vi "Run_Core.vi"(0 "Message Popup in":refnum<class "ControllerData.lvclass">, 11 "error in (no error)":errorcluster) -> (4 "Message Popup out":refnum<class "ControllerData.lvclass">, 6 "Return":variant, 15 "error out":errorcluster)   [LabVIEW 2019, in "ControllerData.lvclass"]
uses:
  ControllerData.lvclass
  ControllerData.lvclass/ControllerData.ctl
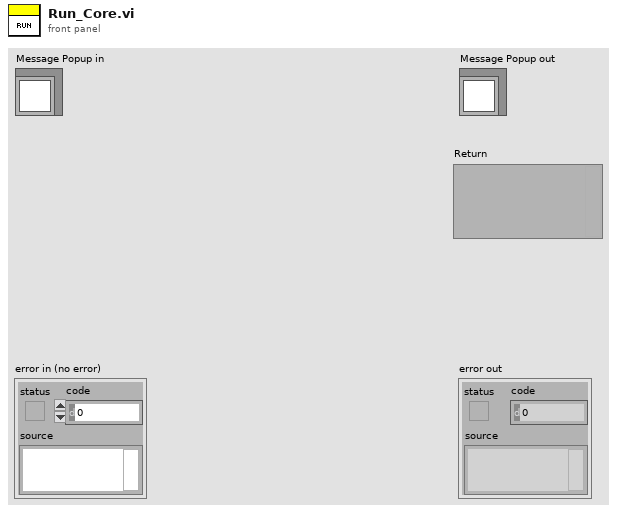
[diagram p1: front panel]
types:
  T1 = typedef "ControllerData.lvclass/Function List.ctl" = enum16{"GetTempTrend", "GetStatus"}
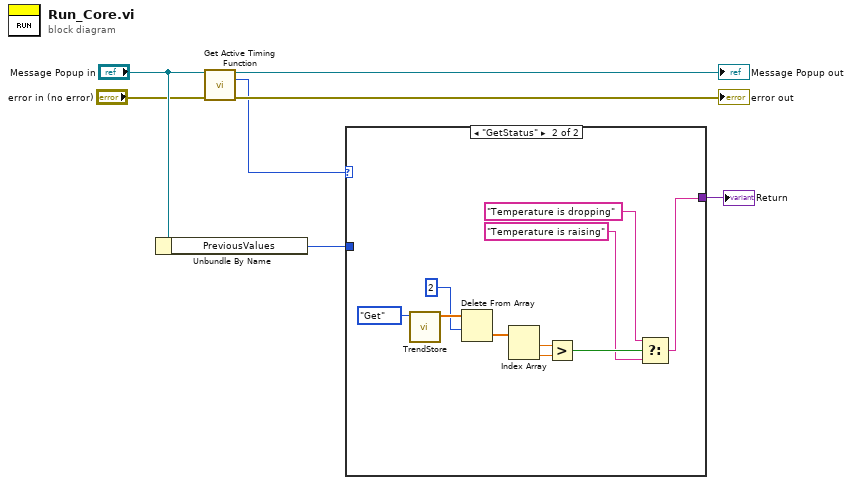
[diagram p0: block diagram]
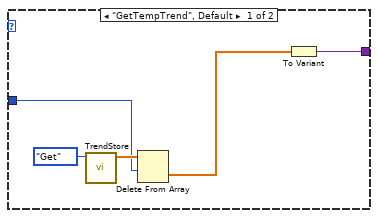
[diagram p2: hidden frame]
diagram:
  n1 = Unbundle By Name("Message Popup in") -> ("PreviousValues"=w7:i32)
  n2 = call "Get Active Timing Function.vi"("Timing Functions in"="Message Popup in", "error in (no error)"="error in (no error)") -> ("Timing Functions out"=→"Message Popup out":refnum<class "ControllerData.lvclass">, "Function List"=w2:T1, "error out"=→"error out":errorcluster)  [unwired: 11 in]
  n3 = case shown="\"GetStatus\"" w2 {
    tunnel: w7 -> [w10 _]
    tunnel: [w8 w13] -> w1
    frame "GetTempTrend", Default {
      n4 = call "TrendStore.vi"("Selector"=enum16{"Init", "Store", "Get"}."Get") -> ("Temperature Trend"=w11:dbl[])  [unwired: 10 in]
      n5 = Delete From Array(array=w11, length=w10) -> (deleted portion=w9:dbl[])  [unwired: 1 in, 1 out]
      n6 = To Variant(anything=w9) -> (Variant=w8:variant)
    }
    frame "GetStatus" {
      n7 = call "TrendStore.vi"("Selector"=enum16{"Init", "Store", "Get"}."Get") -> ("Temperature Trend"=w22:dbl[])  [unwired: 10 in]
      n8 = Delete From Array(array=w22, length=2) -> (deleted portion=w19:dbl[])  [unwired: 1 in, 1 out]
      n9 = Index Array(array=w19) -> (element #1=w17:dbl, element #2=w18:dbl)  [unwired: 2 in]
      n10 = Greater?(x=w17, y=w18) -> (0:w16:bool)
      n11 = Select(t="Temperature is dropping", s=w16, f="Temperature is raising") -> (s? t:f=w13:string)
    }
  }
  "Return" <- w1
